vi "variablesglobales.vi"() -> ()   [LabVIEW 2018]
panel:
  out "salida":string
  out "entrada":string
  out "Arreglo_recibido":dbl[](array[numeric])
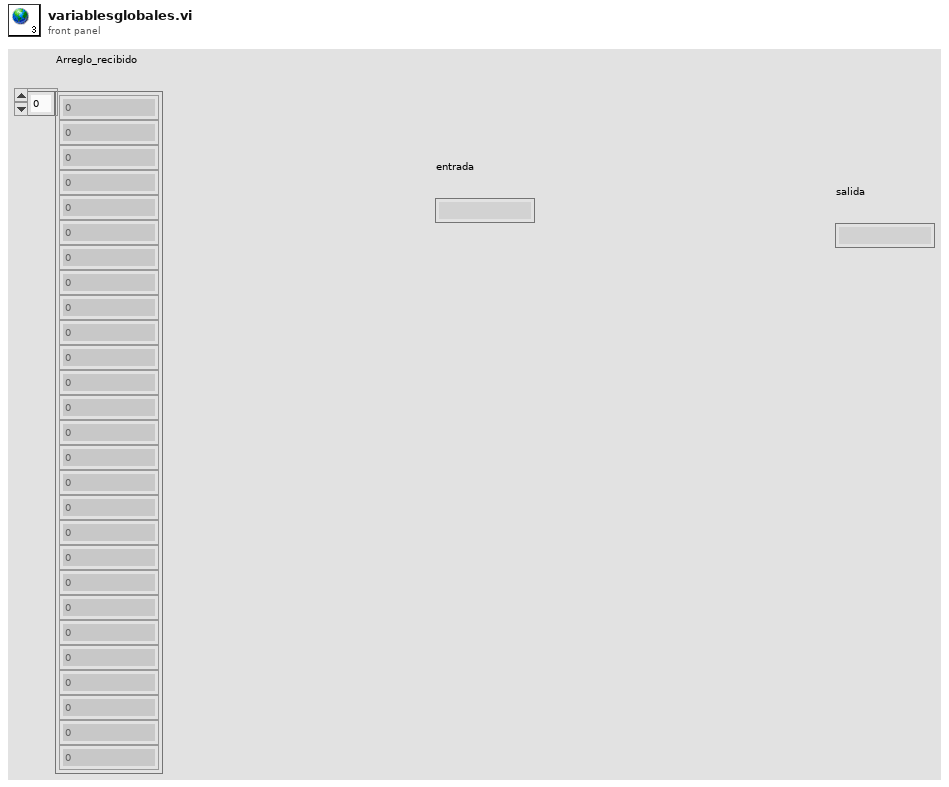
[diagram p1: front panel]
diagram:
